vi "WLAN Fetch SEM.vi"(0 "Instrument Handle In":refnum<k21>, 1 "Selector String":string, 11 "error in (no error)":errorcluster) -> (4 "Instrument Handle Out":refnum<k21>, 6 "WLAN SEM Results":T1 {"Upper Offset Margin Relative Power (dB)" format="%.2f"; "Upper Offset Margin Absolute Power (dBm)" format="%.2f"; "Upper Offset Margin Frequency (Hz)" format="%.3p"; "Upper Offset Margin (dB)" format="%.2f"; "Upper Offset Measurement Status" items=["Fail", "Pass"]; "Lower Offset Margin Relative Power (dB)" format="%.2f"; "Lower Offset Margin Absolute Power (dBm)" format="%.2f"; "Lower Offset Margin Frequency (Hz)" format="%.3p"; "Lower Offset Margin (dB)" format="%.2f"; "Lower Offset Measurement Status" items=["Fail", "Pass"]; "Relative Power (dB)" format="%.2f"; "Absolute Power (dBm)" format="%.2f"; "Measurement Status" items=["Fail", "Pass"]}, 15 "error out":errorcluster)   [LabVIEW 2016, in "RFmxWLAN.lvlib"]
uses:
  RFmxWLAN.lvlib
  Typedefs/WLAN SEM Results.ctl
  <vilib>/RFmx/WLAN/mx/RFmxWLAN.llb/RFmxWLAN SEM Fetch Measurement Status.vi
  <vilib>/RFmx/WLAN/mx/RFmxWLAN.llb/RFmxWLAN SEM Fetch Carrier Measurement.vi
  <vilib>/RFmx/WLAN/mx/RFmxWLAN.llb/RFmxWLAN SEM Fetch Lower Offset Margin (Array).vi
  <vilib>/RFmx/WLAN/mx/RFmxWLAN.llb/RFmxWLAN SEM Fetch Upper Offset Margin (Array).vi
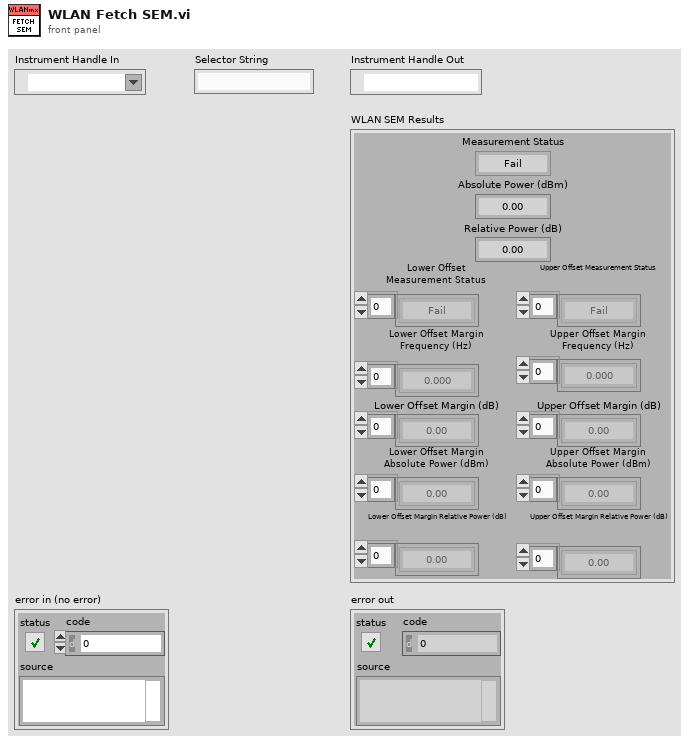
[diagram p1: front panel]
types:
  T1 = typedef "RFmxWLAN.lvlib/WLAN SEM Results.ctl" = cluster{"Measurement Status":i32, "Absolute Power (dBm)":dbl, "Relative Power (dB)":dbl, "Lower Offset Measurement Status":i32[], "Lower Offset Margin (dB)":dbl[], "Lower Offset Margin Frequency (Hz)":dbl[], "Lower Offset Margin Absolute Power (dBm)":dbl[], "Lower Offset Margin Relative Power (dB)":dbl[], "Upper Offset Measurement Status":i32[], "Upper Offset Margin (dB)":dbl[], "Upper Offset Margin Frequency (Hz)":dbl[], "Upper Offset Margin Absolute Power (dBm)":dbl[], "Upper Offset Margin Relative Power (dB)":dbl[]}
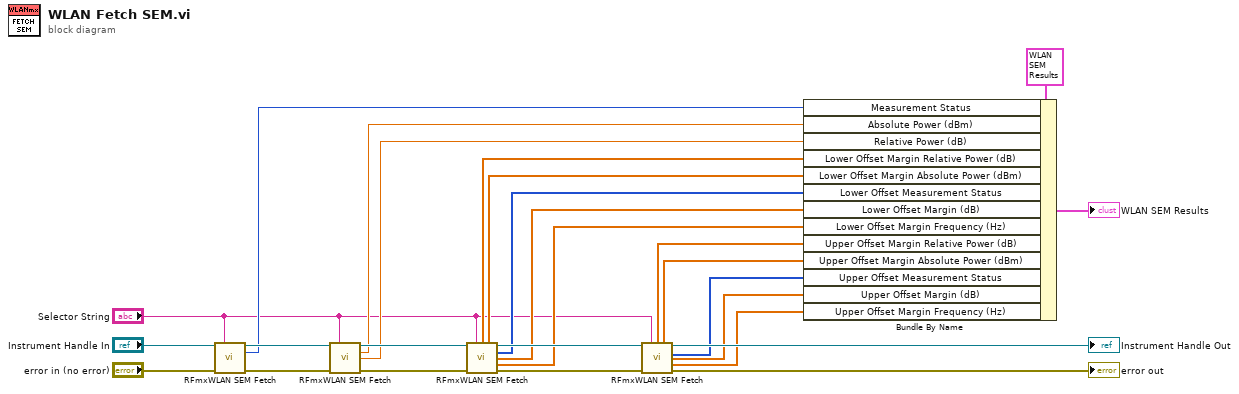
[diagram p0: block diagram]
diagram:
  n1 = call-poly <vilib>:"RFmxWLAN SEM Fetch.vi"("Instrument Handle In"="Instrument Handle In", "Selector String"="Selector String", "error in (no error)"="error in (no error)") -> ("Instrument Handle Out"=w22:refnum<k21>, "Measurement Status"=w15:i32, "error out"=w25:errorcluster)  [unwired: 10 in]
  n2 = call-poly <vilib>:"RFmxWLAN SEM Fetch.vi"("Instrument Handle In"=w22, "Selector String"="Selector String", "error in (no error)"=w25) -> ("Instrument Handle Out"=w20:refnum<k21>, "Absolute Power (dBm)"=w14:dbl, "Relative Power (dB)"=w13:dbl, "error out"=w23:errorcluster)  [unwired: 9 in]
  n3 = call-poly <vilib>:"RFmxWLAN SEM Fetch.vi"("Instrument Handle In"=w20, "Selector String"="Selector String", "error in (no error)"=w23) -> ("Margin Relative Power (dB)"=w12:dbl[], "Margin Absolute Power (dBm)"=w11:dbl[], "Instrument Handle Out"=w18:refnum<k21>, "Measurement Status"=w10:i32[], "Margin (dB)"=w9:dbl[], "Margin Frequency (Hz)"=w8:dbl[], "error out"=w21:errorcluster)  [unwired: 6 in]
  n4 = call-poly <vilib>:"RFmxWLAN SEM Fetch.vi"("Instrument Handle In"=w18, "Selector String"="Selector String", "error in (no error)"=w21) -> ("Margin Relative Power (dB)"=w7:dbl[], "Margin Absolute Power (dBm)"=w6:dbl[], "Instrument Handle Out"=→"Instrument Handle Out":refnum<k21>, "Measurement Status"=w5:i32[], "Margin (dB)"=w4:dbl[], "Margin Frequency (Hz)"=w3:dbl[], "error out"=→"error out":errorcluster)  [unwired: 6 in]
  n5 = Bundle By Name(cluster=T1 {"Measurement Status"=0, "Absolute Power (dBm)"=0.0, "Relative Power (dB)"=0.0, "Lower Offset Measurement Status"=[], "Lower Offset Margin (dB)"=[], "Lower Offset Margin Frequency (Hz)"=[], "Lower Offset Margin Absolute Power (dBm)"=[], "Lower Offset Margin Relative Power (dB)"=[], "Upper Offset Measurement Status"=[], "Upper Offset Margin (dB)"=[], "Upper Offset Margin Frequency (Hz)"=[], "Upper Offset Margin Absolute Power (dBm)"=[], "Upper Offset Margin Relative Power (dB)"=[]} ("Cluster"), "Measurement Status"=w15, "Absolute Power (dBm)"=w14, "Relative Power (dB)"=w13, "Lower Offset Margin Relative Power (dB)"=w12, "Lower Offset Margin Absolute Power (dBm)"=w11, "Lower Offset Measurement Status"=w10, "Lower Offset Margin (dB)"=w9, "Lower Offset Margin Frequency (Hz)"=w8, "Upper Offset Margin Relative Power (dB)"=w7, "Upper Offset Margin Absolute Power (dBm)"=w6, "Upper Offset Measurement Status"=w5, "Upper Offset Margin (dB)"=w4, "Upper Offset Margin Frequency (Hz)"=w3) -> (→"WLAN SEM Results":T1)
